vi "Pretrigger Buffer (by ref).vi"(5 "Mode":enum16{"Initialize", "Add", "Read"}(ring), 7 "Pretrigger Length":i32, 8 "# Channels":i32, 10 "New Data":sgl[](array[numeric])) -> (0 "Current Size":i32, 2 "Pretrigger Data":sgl[][](array[numeric]))   [LabVIEW 2023]
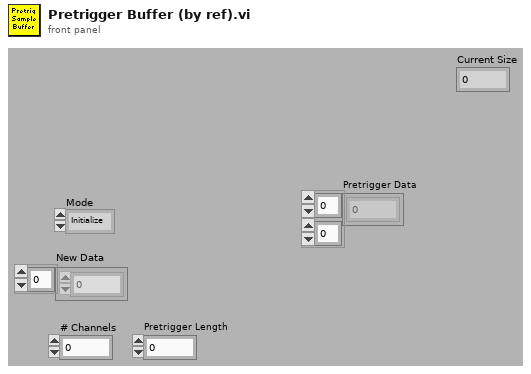
[diagram p1: front panel]
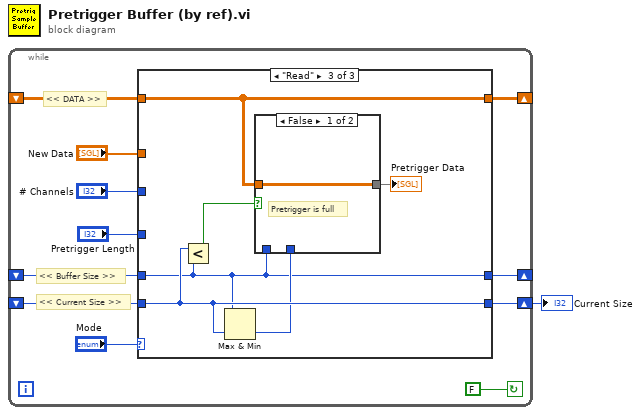
[diagram p0: block diagram]
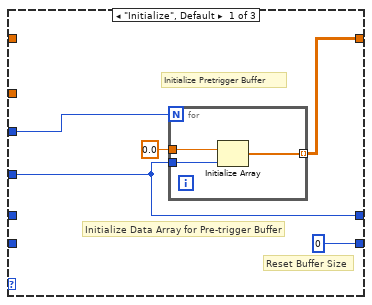
[diagram p2: hidden frame]
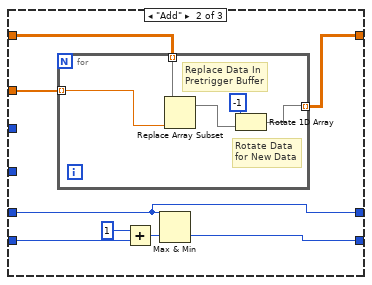
[diagram p3: hidden frame]
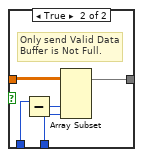
[diagram p4: hidden frame]
diagram:
  n1 = while {
    shift-right: [w6] -> _
    shift-left: _ -> [w11]
    shift-right: [w8] -> w1
    shift-left: _ -> [w3]
    shift-right: [w5] -> _
    shift-left: _ -> [w4]
    stop <- FALSE continue-if-true
    # "<< Buffer Size >>"
    # "<< Current Size >>"
    # "<< DATA >>"
    n2 = case shown="\"Read\"" "Mode" {
      tunnel: w11 -> [_ w28 w38]
      tunnel: "# Channels" -> [w16 _ _]
      tunnel: "New Data" -> [_ w26 _]
      tunnel: [0 w22 w36] -> w8
      tunnel: "Pretrigger Length" -> [w14 _ _]
      tunnel: [w13 w27 w38] -> w6
      tunnel: [w14 w23 w34] -> w5
      tunnel: w4 -> [_ w23 w34]
      tunnel: w3 -> [_ w24 w36]
      frame "Initialize", Default {
        # "Reset Buffer Size"
        # "Initialize Pretrigger Buffer"
        # "Initialize Data Array for Pre-trigger Buffer"
        n3 = for {
          N: w16 -> [_]
          tunnel: sgl 0.0 ("element") -> [w20]
          tunnel: w14 -> [w19]
          tunnel: [w18] -> w13 mode=indexing
          n4 = Initialize Array(w20, w19) -> (w18:sgl[])
        }
      }
      frame "Add" {
        n5 = for {
          tunnel: w28 -> [w33] mode=indexing
          tunnel: [w31] -> w27 mode=indexing
          tunnel: w26 -> [w30] mode=indexing
          # "Rotate Data\nfor New Data"
          # "Replace Data In \nPretrigger Buffer"
          n6 = Replace Array Subset(array=w33, new element=w30) -> (w32:sgl[])  [unwired: 1 in]
          n7 = Rotate 1D Array(1:w32, 2:-1 ("n")) -> (0:w31:sgl[])
        }
        n8 = Add(x=1, y=w24) -> (x+y=w25:i32)
        n9 = Max & Min(x=w23, y=w25) -> (min(x,y)=w22:i32)  [unwired: 1 out]
      }
      frame "Read" {
        n10 = Less?(x=w36, y=w34) -> (x < y?=w39:bool)
        n11 = Max & Min(x=w34, y=w36) -> (min(x,y)=w35:i32)  [unwired: 1 out]
        n12 = case shown="False" w39 {
          tunnel: w38 -> [w40 w45]
          tunnel: [w40 w44] -> w37
          tunnel: w35 -> [_ w42]
          tunnel: w34 -> [_ w41]
          frame False {
            # "Pretrigger is full"
          }
          frame True {
            # "Only send Valid Data\nBuffer is Not Full."
            n13 = Subtract(x=w41, y=w42) -> (x-y=w43:i32)
            n14 = Array Subset(array=w45, index (col)=w43, length (col)=w42) -> (w44:sgl[][])  [unwired: 2 in]
          }
        }
        "Pretrigger Data" <- w37
      }
    }
  }
  "Current Size" <- w1
